vi "Time.Time of Day to Today Time.vi"(11 "Time Of Day":timestamp format="%<%I:%M:%S %p>T") -> (2 "Past":bool, 3 "Time Today":timestamp)   [LabVIEW 2019]
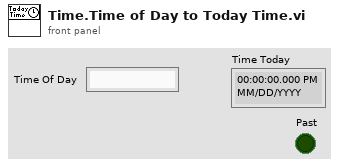
[diagram p1: front panel]
types:
  T1 = typedef "LVDateTimeRec.ctl" = cluster{"fractional second":dbl, "second":i32, "minute":i32, "hour":i32, "day of month":i32, "month":i32, "year":i32, "day of week":i32, "day of year":i32, "DST":i32}
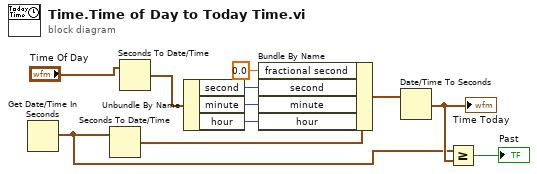
[diagram p0: block diagram]
diagram:
  n1 = Get Date/Time In Seconds() -> (seconds since 1Jan1904=w1:timestamp)
  n2 = Seconds To Date/Time(time stamp (now)=w1) -> (date time rec=w10:T1)  [unwired: 1 in]
  n3 = Seconds To Date/Time(time stamp (now)="Time Of Day") -> (date time rec=w9:T1)  [unwired: 1 in]
  n4 = Unbundle By Name(w9) -> ("second"=w8:i32, "minute"=w7:i32, "hour"=w6:i32)
  n5 = Bundle By Name(cluster=w10, "fractional second"=0.0, "second"=w8, "minute"=w7, "hour"=w6) -> (w4:T1)
  n6 = Date/Time To Seconds(2:w4) -> (0:w2:timestamp)  [unwired: 1 in]
  "Time Today" <- w2
  n7 = Greater Or Equal?(x=w1, y=w2) -> (x >= y?=→"Past":bool)
